vi "Toggle Button.vi"(1 "Input":bool=TRUE) -> (0 "Output":bool)   [LabVIEW 2012]
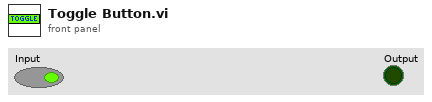
[diagram p1: front panel]
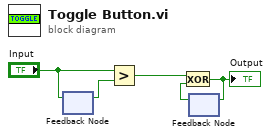
[diagram p0: block diagram]
diagram:
  n1 = feedback-in #1("Input") -> ()
  n2 = feedback #1() -> (w2:bool)  [unwired: 1 in]
  n3 = Greater?(x="Input", y=w2) -> (0:w5:bool)
  n4 = feedback #2() -> (w3:bool)  [unwired: 1 in]
  n5 = Exclusive Or(1:w3, 2:w5) -> (0:w4:bool)
  "Output" <- w4
  n6 = feedback-in #2(w4) -> ()
